vi "Slit.vi"(8 "error in (no error)":errorcluster, 10 "Notifiers":T1, 11 "All Message Queue Cluster":T2) -> (0 "error out":errorcluster)   [LabVIEW 2013]
doc: "Ce VI est la partie visualisation des Fentes. Elle permet l'envoie d'ordre à cette appareil et affiche son état.\n- Connected : indique si l'appareil est connecté.\n- Open : indique l'ouverture de la fente.\n- Status : indique le status actuel de la fente. CAD s'il y a une erreur, ou si elle est en mouvement, etc ..."
uses:
  Lib QMH/AllMessageQueue Cluster.ctl
  Lib QMH/Message Cluster.ctl
  Lib Notifier/Notifier.ctl
  Slit UI data.ctl
  Slit config.ctl
  FGV/Action Slit.ctl
  FGV/FGV Slit Data.ctl
  Lib IHM Control/Front Panel Status.ctl
  support/Status.vi
  Lib QMH/MessageQueues.lvlib
  Lib IHM Control/IHM Control.lvlib
  Lib Notifier/Notifier.lvlib
panel:
  out "Opening":dbl format="%#_3g"
  out "Connected":bool
  out "Status":string
  # "Slit"
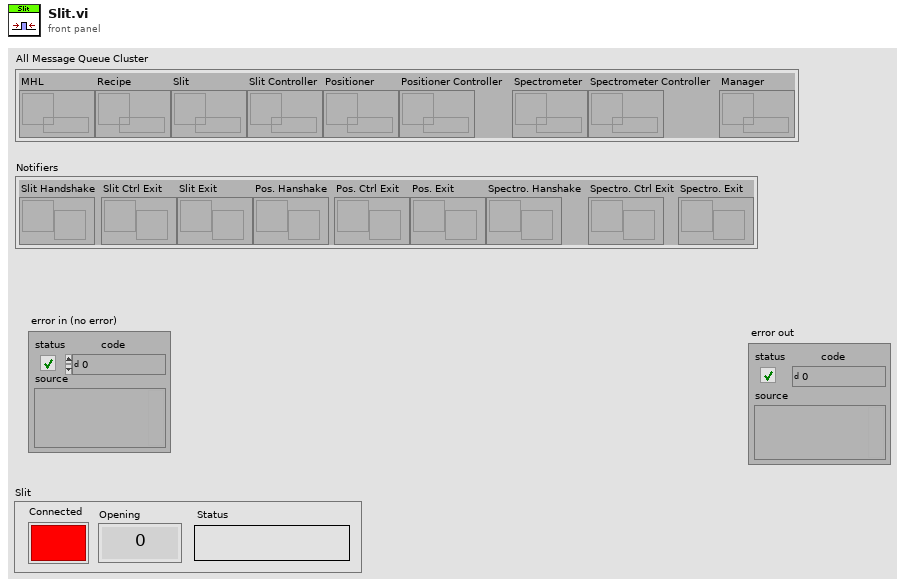
[diagram p1: front panel]
types:
  T1 = typedef "Notifier.lvlib/Notifier.ctl" = cluster{"Slit Handshake":refnum<notifier>, "Slit Ctrl Exit":refnum<notifier>, "Slit Exit":refnum<notifier>, "Pos. Hanshake":refnum<notifier>, "Pos. Ctrl Exit":refnum<notifier>, "Pos. Exit":refnum<notifier>, "Spectro. Hanshake":refnum<notifier>, "Spectro. Ctrl Exit":refnum<notifier>, "Spectro. Exit":refnum<notifier>}
  T2 = typedef "MessageQueues.lvlib/AllMessageQueue Cluster.ctl" = cluster{"MHL":refnum<queue>, "Recipe":refnum<queue>, "Slit":refnum<queue>, "Slit Controller":refnum<queue>, "Positioner":refnum<queue>, "Positioner Controller":refnum<queue>, "Spectrometer":refnum<queue>, "Spectrometer Controller":refnum<queue>, "Manager":refnum<queue>}
  T3 = typedef "Slit config.ctl" = cluster{"VISA resource name":refnum<visa-resource-name>}
  T4 = typedef "Slit UI data.ctl" = cluster{"Connected":bool, "Status":string, "Openning":dbl}
  T5 = typedef "Action Slit.ctl" = enum16{"Connect", "Initialize", "Set Velocity", "Get Velocity", "Move Rel", "Move Abs", "Position", "Status", "Abort", "Disconnect"}
  T6 = typedef "FGV Slit Data.ctl" = cluster{"Portnumber":i32, "Position":dbl, "Status":string, "Système ID":i32, "Connected axes":string[], "Velocity":dbl, "Stage names":string[], "Device ID out":i32}
  T7 = typedef "IHM Control.lvlib/Front Panel Status.ctl" = enum16{"Initialisation", "Enable Slit", "Enable Positionner", "Enable Spectrometer", "Disable Slit", "Disable Positionner", "Disable Spectrometer"}
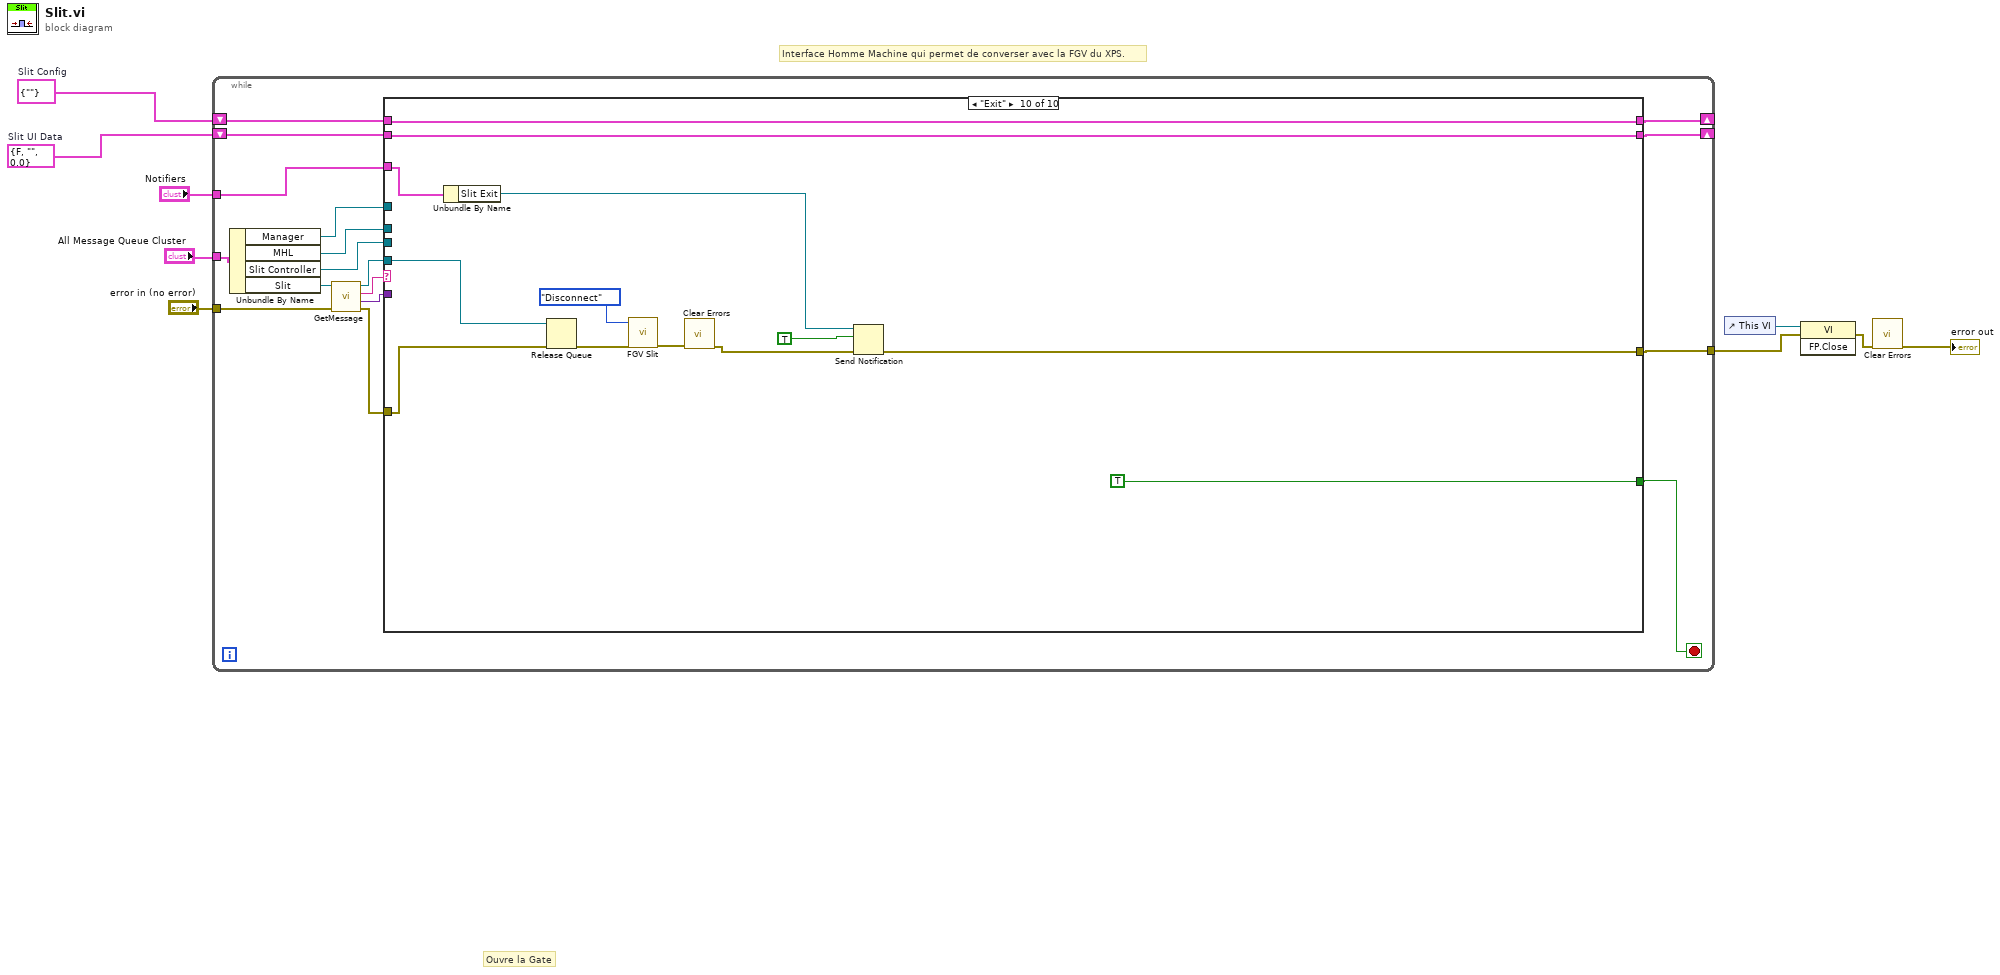
[diagram p0: block diagram]
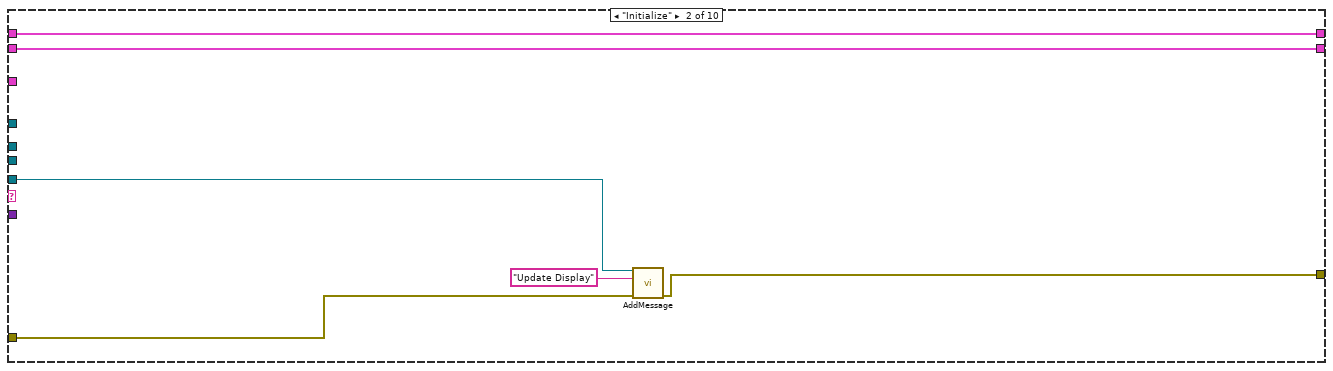
[diagram p3: hidden frame]
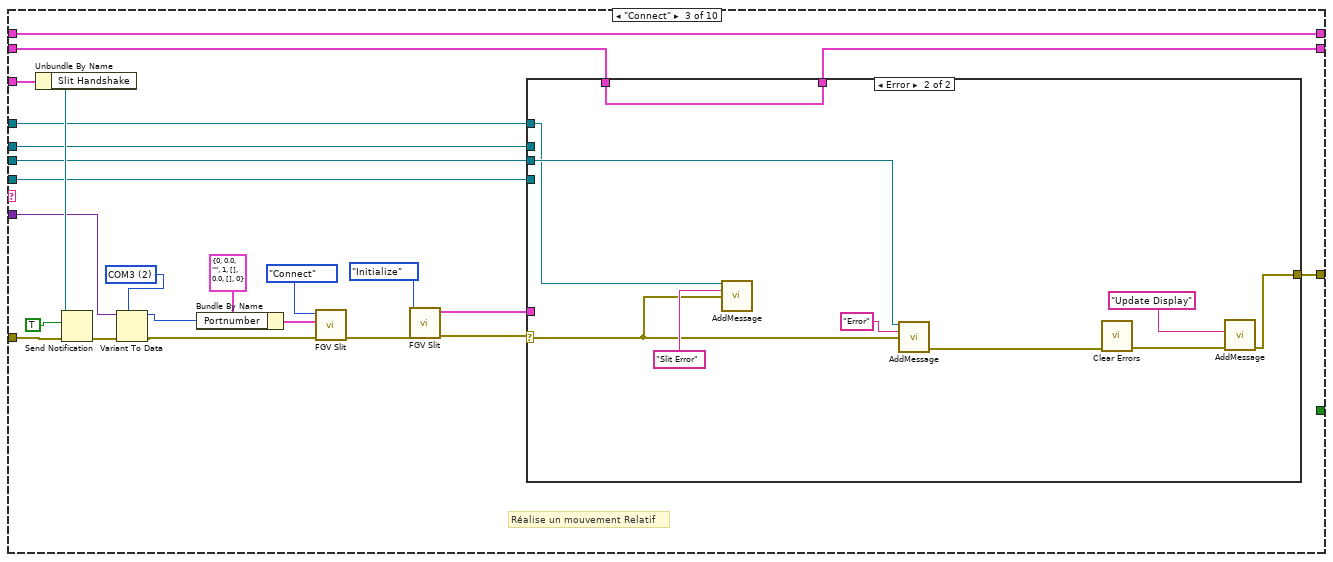
[diagram p4: hidden frame]
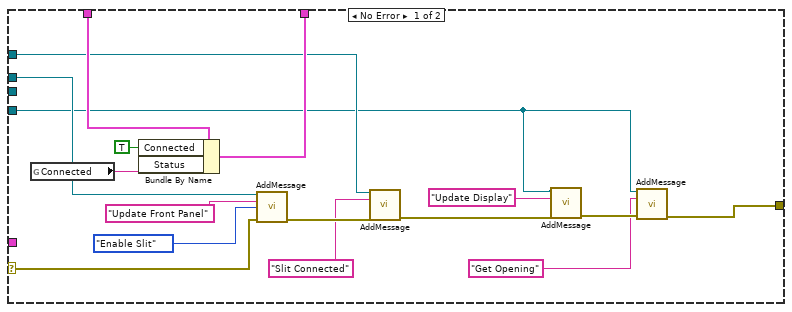
[diagram p5: hidden frame]
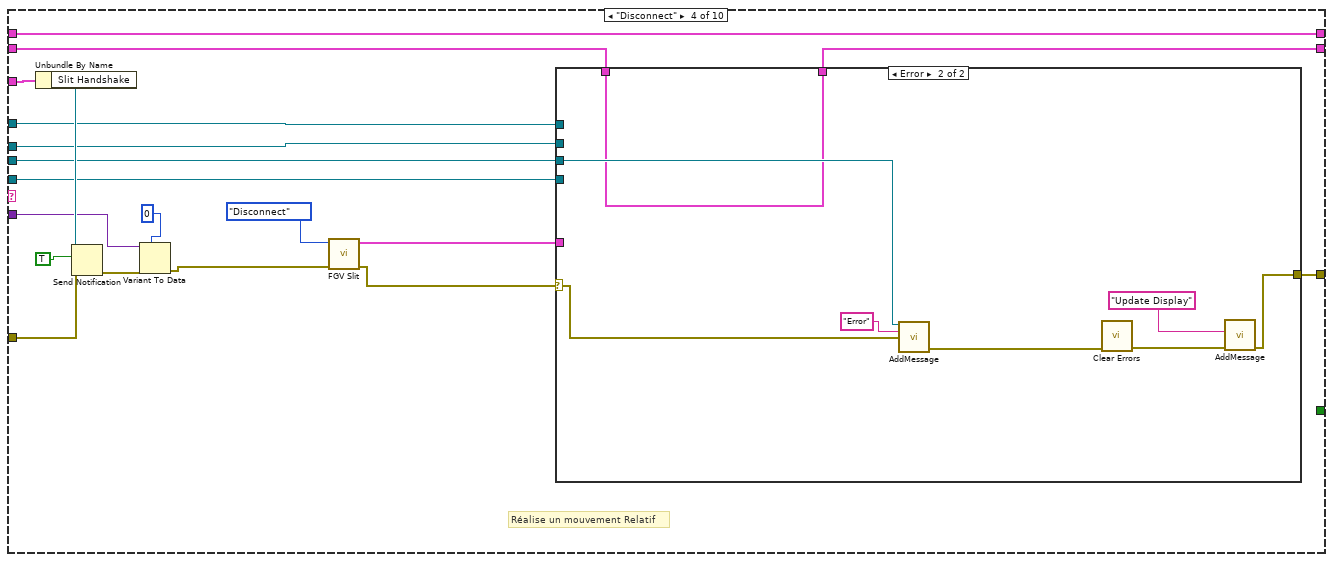
[diagram p6: hidden frame]
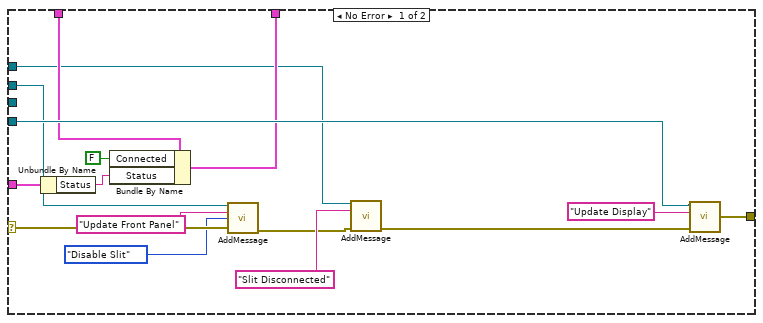
[diagram p7: hidden frame]
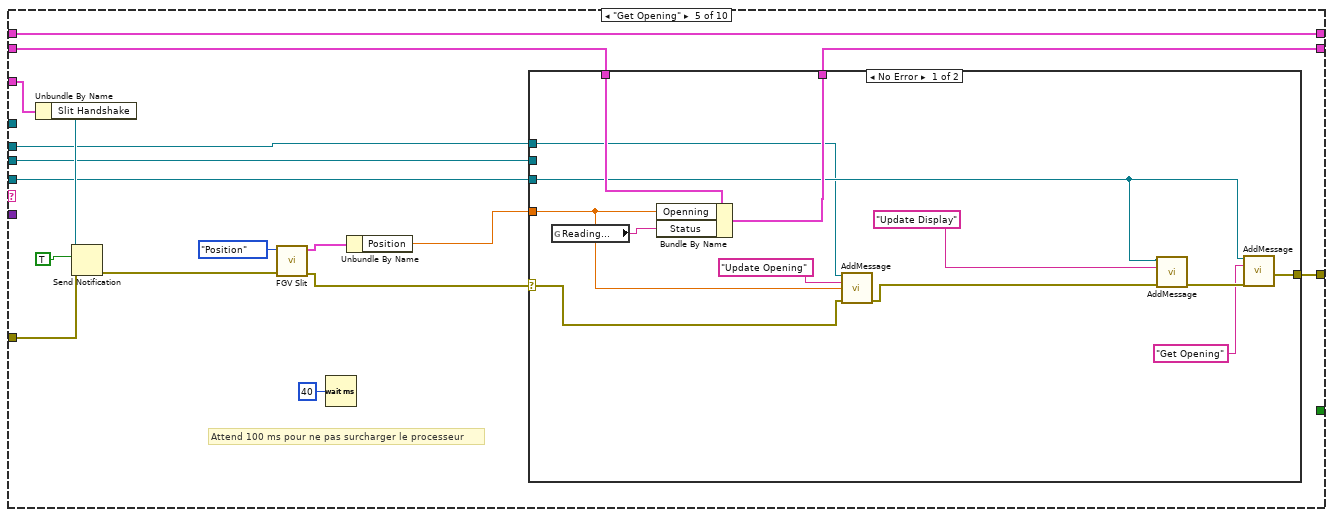
[diagram p8: hidden frame]
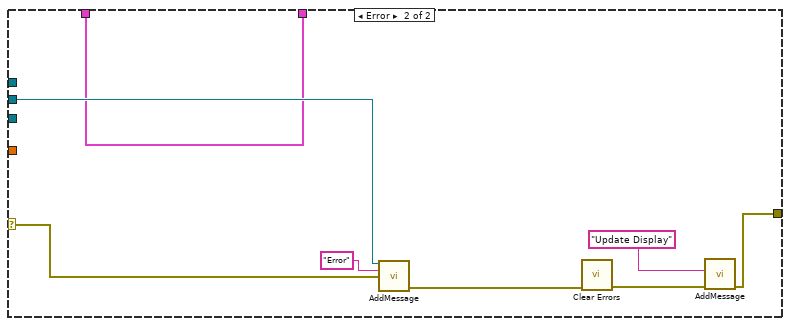
[diagram p9: hidden frame]
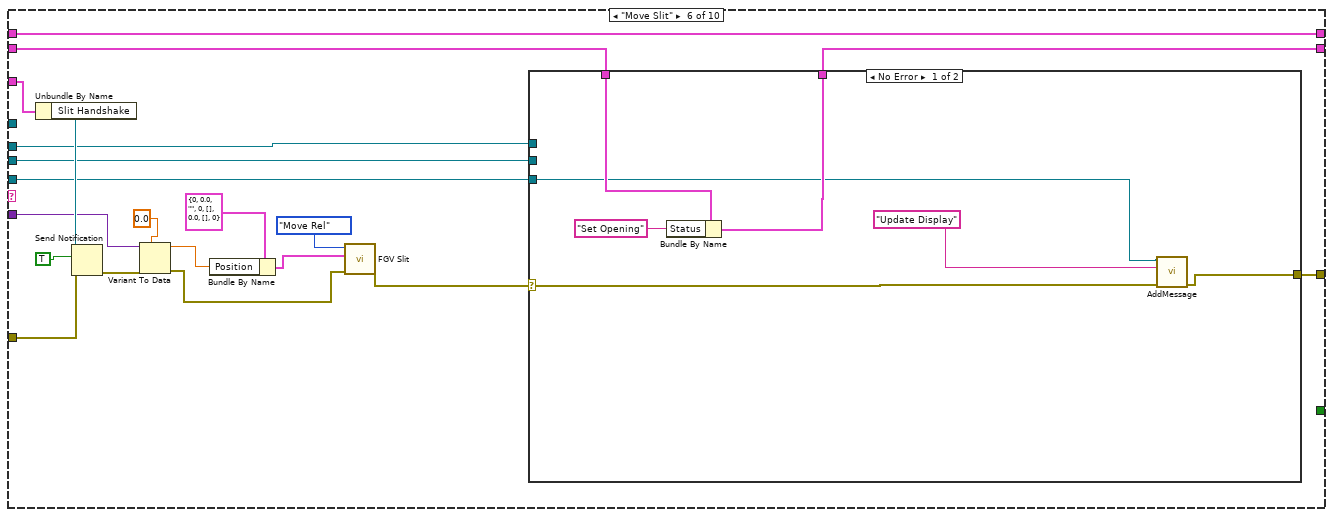
[diagram p10: hidden frame]
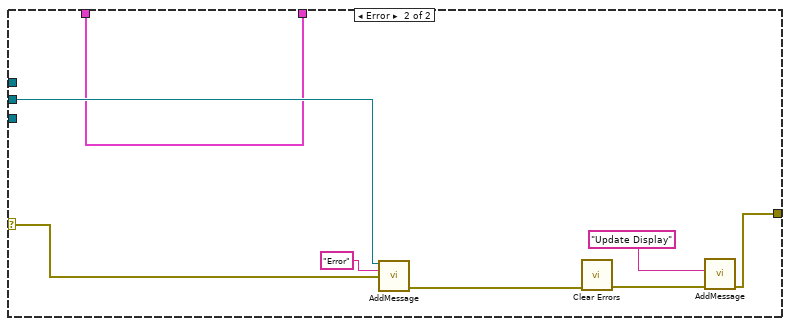
[diagram p11: hidden frame]
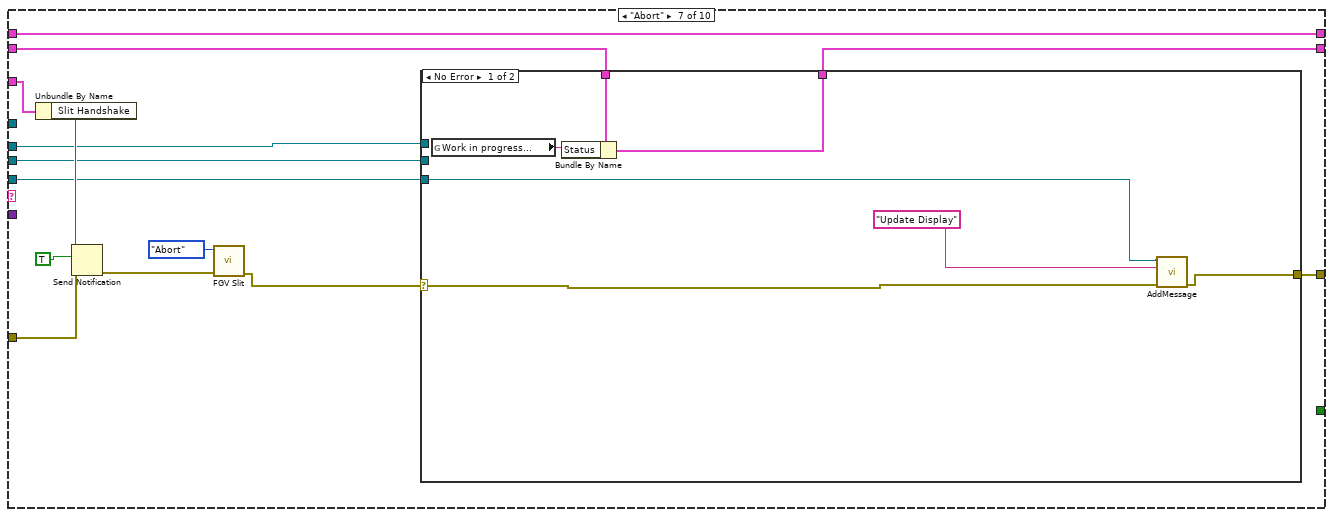
[diagram p12: hidden frame]
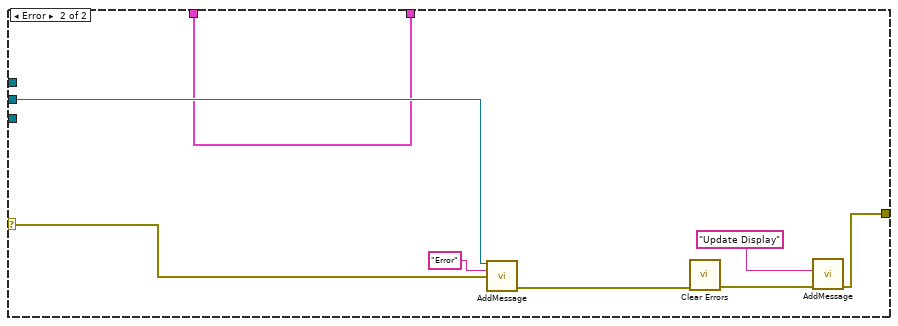
[diagram p13: hidden frame]
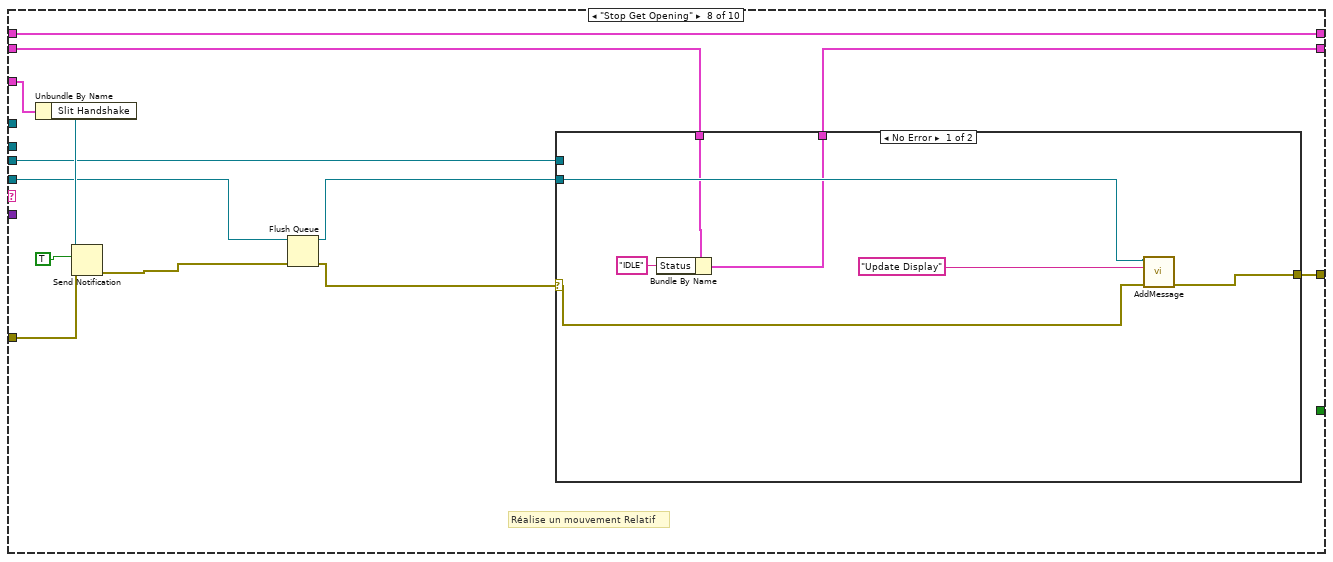
[diagram p14: hidden frame]
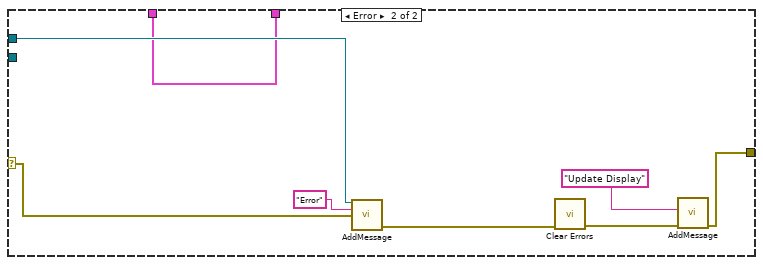
[diagram p15: hidden frame]
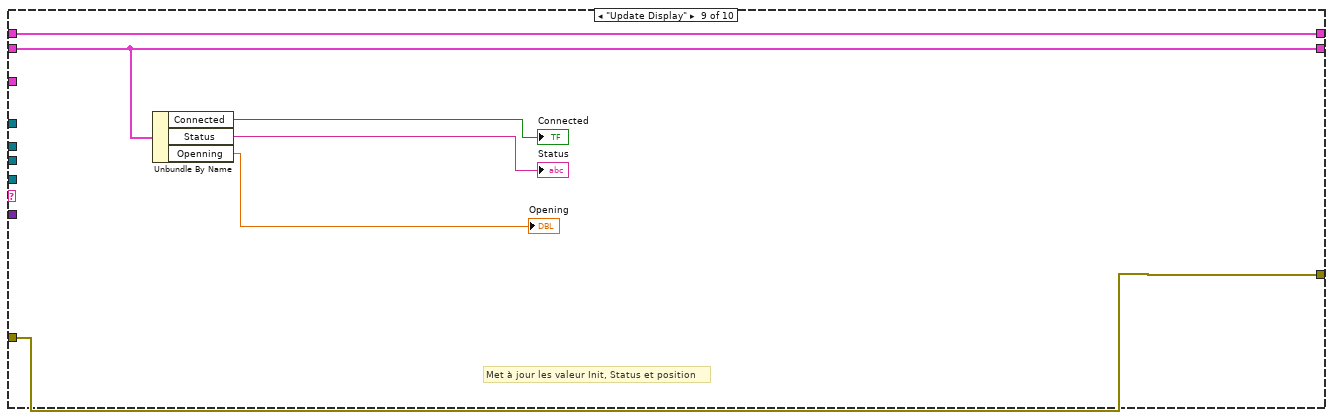
[diagram p16: hidden frame]
diagram:
  w5 = T3 {"VISA resource name"=""}  # Slit Config
  w6 = T4 {"Connected"=FALSE, "Status"="", "Openning"=0.0}  # Slit UI Data
  # "Interface Homme Machine qui permet de converser avec la FGV du XPS."
  # "Ouvre la Gate"
  n1 = while {
    tunnel: "All Message Queue Cluster" -> [w24]
    tunnel: "Notifiers" -> [w17]
    tunnel: "error in (no error)" -> [w25]
    tunnel: [w19] -> w2
    shift-right: [w21] -> _
    shift-left: w5 -> [w23]
    shift-right: [w20] -> _
    shift-left: w6 -> [w22]
    stop <- w18 stop-if-true
    n2 = Unbundle By Name(w24) -> ("Manager"=w16:refnum<queue>, "MHL"=w15:refnum<queue>, "Slit Controller"=w14:refnum<queue>, "Slit"=w26:refnum<queue>)
    n3 = call "GetMessage.vi"("entrée d'erreur"=w25, "Message queue"=w26) -> ("sortie d'erreur"=w12:errorcluster, "Data"=w11:variant, "Message"=w10:string, "Dup Message Queue"=w13:refnum<queue>)  [unwired: 6 in]
    n4 = case shown="\"Exit\"" w10 {
      tunnel: w17 -> [_ _ w57 w103 w144 w185 w214 w242 _ w277]
      tunnel: w13 -> [_ w30 w56 w102 w143 w184 w213 w234 _ w271]
      tunnel: w11 -> [_ _ w43 w94 _ w177 _ _ _ _]
      tunnel: w12 -> [w29 w32 w50 w96 w138 w179 w208 w236 w264 w272]
      tunnel: [w29 w31 w55 w101 w142 w183 w212 w241 w264 w274] -> w19
      tunnel: w14 -> [_ _ w54 w100 w141 w182 w211 w240 _ _]
      tunnel: [_ _ _ _ _ _ _ _ _ TRUE] -> w18
      tunnel: w23 -> [w28 w35 w53 w99 w140 w181 w210 w239 w265 w273]
      tunnel: [w28 w35 w53 w99 w140 w181 w210 w239 w265 w273] -> w21
      tunnel: w22 -> [w27 w34 w52 w98 w135 w174 w206 w238 w263 w270]
      tunnel: [w27 w34 w51 w97 w139 w180 w209 w237 w263 w270] -> w20
      tunnel: w15 -> [_ _ w49 w92 w136 w175 w207 _ _ _]
      tunnel: w16 -> [_ _ w48 w91 _ _ _ _ _ _]
      frame Default {
        # "ne fait rien si le message dépilé n'existe pas"
      }
      frame "Initialize" {
        n5 = call "AddMessage.vi"("Message queue"=w30, "Message"="Update Display", "entrée d'erreur (pas d'erreur)"=w32) -> ("error out"=w31:errorcluster)  [unwired: 11 in, 1 out]
      }
      frame "Connect" {
        w42 = 2 items=["COM1", "COM2", "COM3", "COM4", "COM5", "COM6", "COM7", "COM8", "COM9", "COM10", "COM11", "COM12", "COM13", "COM14", "COM15", "COM16", "COM17", "COM18", "COM19", "COM20", "COM21", "COM22", "COM23", "COM24", "COM25", "COM26", "COM27", "COM28", "COM29", "COM30"] ("Portnumber")
        # "Réalise un mouvement Relatif"
        n6 = Unbundle By Name(w57) -> ("Slit Handshake"=w59:refnum<notifier>)
        n7 = Send Notification(notification=TRUE, notifier=w59, error in (no error)=w50) -> (error out=w44:errorcluster)  [unwired: 1 out]
        n8 = Variant To Data(error in=w44, type=w42, Variant=w43) -> (data=w40:i32, error out=w41:errorcluster)
        n9 = Bundle By Name(cluster=T6 {"Portnumber"=0, "Position"=0.0, "Status"="", "Système ID"=1, "Connected axes"=[], "Velocity"=0.0, "Stage names"=[], "Device ID out"=0} ("FGV Slit Data"), "Portnumber"=w40) -> (w45:T6)
        n10 = call "FGV Slit.vi"("error in (no error)"=w41, "FGV Slit Data In"=w45, "Action"=Action_Slit."Connect") -> ("error out"=w39:errorcluster)  [unwired: 7 in, 1 out]
        n11 = call "FGV Slit.vi"("error in (no error)"=w39, "Action"=Action_Slit."Initialize") -> ("error out"=w38:errorcluster, "FGV Slit Data Out"=w36:T6)  [unwired: 8 in]
        n12 = case shown="Error" w38 {
          selector: w38 -> [w72 w77]
          tunnel: w56 -> [w61 _]
          tunnel: [w62 w82] -> w55
          tunnel: w54 -> [_ w81]
          tunnel: w52 -> [w75 w80]
          tunnel: [w74 w80] -> w51
          tunnel: w49 -> [w71 _]
          tunnel: w48 -> [w66 w78]
          tunnel: w36 -> [_ _]
          frame No Error {
            n13 = global read "Status.vi" "Connected"() -> (w64:string)
            n14 = Bundle By Name(cluster=w75, "Connected"=TRUE, "Status"=w64) -> (w74:T4)
            n15 = call "AddMessage.vi"("Message queue"=w71, "Message"="Update Front Panel", "Data"=Front_Panel_Status."Enable Slit" ("Front Panel status"), "entrée d'erreur (pas d'erreur)"=w72) -> ("error out"=w68:errorcluster)  [unwired: 10 in, 1 out]
            n16 = call "AddMessage.vi"("Message queue"=w66, "Message"="Slit Connected", "entrée d'erreur (pas d'erreur)"=w68) -> ("error out"=w67:errorcluster)  [unwired: 11 in, 1 out]
            n17 = call "AddMessage.vi"("Message queue"=w61, "Message"="Update Display", "entrée d'erreur (pas d'erreur)"=w67) -> ("error out"=w63:errorcluster)  [unwired: 11 in, 1 out]
            n18 = call "AddMessage.vi"("Message queue"=w61, "Message"="Get Opening", "entrée d'erreur (pas d'erreur)"=w63) -> ("error out"=w62:errorcluster)  [unwired: 11 in, 1 out]
          }
          frame Error {
            n19 = call "AddMessage.vi"("Message queue"=w78, "Message"="Slit Error", "Data"=w77) -> ()  [unwired: 11 in, 2 out]
            n20 = call "AddMessage.vi"("Message queue"=w81, "Message"="Error", "Data"=w77) -> ("error out"=w85:errorcluster)  [unwired: 11 in, 1 out]
            n21 = call <vilib>:"Clear Errors.vi"("error in (no error)"=w85) -> ("error out"=w83:errorcluster)  [unwired: 6 in]
            n22 = call "AddMessage.vi"("Message"="Update Display", "entrée d'erreur (pas d'erreur)"=w83) -> ("error out"=w82:errorcluster)  [unwired: 12 in, 1 out]
          }
        }
      }
      frame "Disconnect" {
        # "Réalise un mouvement Relatif"
        n23 = Unbundle By Name(w103) -> ("Slit Handshake"=w105:refnum<notifier>)
        n24 = Send Notification(notification=TRUE, notifier=w105, error in (no error)=w96) -> (error out=w95:errorcluster)  [unwired: 1 out]
        n25 = Variant To Data(error in=w95, type=0, Variant=w94) -> (error out=w90:errorcluster)  [unwired: 1 out]
        n26 = call "FGV Slit.vi"("error in (no error)"=w90, "Action"=Action_Slit."Disconnect") -> ("error out"=w89:errorcluster, "FGV Slit Data Out"=w87:T6)  [unwired: 8 in]
        n27 = case shown="Error" w89 {
          selector: w89 -> [w115 w124]
          tunnel: w102 -> [w121 _]
          tunnel: [w119 w125] -> w101
          tunnel: w100 -> [_ w123]
          tunnel: w98 -> [w118 w122]
          tunnel: [w117 w122] -> w97
          tunnel: w92 -> [w114 _]
          tunnel: w91 -> [w108 _]
          tunnel: w87 -> [w107 _]
          frame No Error {
            n28 = Unbundle By Name(w107) -> ("Status"=w106:string)
            n29 = Bundle By Name(cluster=w118, "Connected"=FALSE, "Status"=w106) -> (w117:T4)
            n30 = call "AddMessage.vi"("Message queue"=w114, "Message"="Update Front Panel", "Data"=Front_Panel_Status."Disable Slit" ("Front Panel status"), "entrée d'erreur (pas d'erreur)"=w115) -> ("error out"=w110:errorcluster)  [unwired: 10 in, 1 out]
            n31 = call "AddMessage.vi"("Message queue"=w108, "Message"="Slit Disconnected", "entrée d'erreur (pas d'erreur)"=w110) -> ("error out"=w109:errorcluster)  [unwired: 11 in, 1 out]
            n32 = call "AddMessage.vi"("Message queue"=w121, "Message"="Update Display", "entrée d'erreur (pas d'erreur)"=w109) -> ("error out"=w119:errorcluster)  [unwired: 11 in, 1 out]
          }
          frame Error {
            n33 = call "AddMessage.vi"("Message queue"=w123, "Message"="Error", "Data"=w124) -> ("error out"=w128:errorcluster)  [unwired: 11 in, 1 out]
            n34 = call <vilib>:"Clear Errors.vi"("error in (no error)"=w128) -> ("error out"=w126:errorcluster)  [unwired: 6 in]
            n35 = call "AddMessage.vi"("Message"="Update Display", "entrée d'erreur (pas d'erreur)"=w126) -> ("error out"=w125:errorcluster)  [unwired: 12 in, 1 out]
          }
        }
      }
      frame "Get Opening" {
        # "Attend 100 ms pour ne pas surcharger le processeur"
        n36 = Unbundle By Name(w144) -> ("Slit Handshake"=w146:refnum<notifier>)
        n37 = Send Notification(notification=TRUE, notifier=w146, error in (no error)=w138) -> (error out=w134:errorcluster)  [unwired: 1 out]
        n38 = call "FGV Slit.vi"("error in (no error)"=w134, "Action"=Action_Slit."Position") -> ("error out"=w133:errorcluster, "FGV Slit Data Out"=w131:T6)  [unwired: 8 in]
        n39 = Wait (ms)(milliseconds to wait=u32 40) -> ()  [unwired: 1 out]
        n40 = Unbundle By Name(w131) -> ("Position"=w130:dbl)
        n41 = case shown="No Error" w133 {
          selector: w133 -> [w152 w162]
          tunnel: w143 -> [w154 _]
          tunnel: [w155 w163] -> w142
          tunnel: w141 -> [_ w161]
          tunnel: w135 -> [w158 w160]
          tunnel: [w157 w160] -> w139
          tunnel: w136 -> [w150 _]
          tunnel: w130 -> [w148 _]
          frame No Error {
            n42 = global read "Status.vi" "Reading..."() -> (w147:string)
            n43 = Bundle By Name(cluster=w158, "Openning"=w148, "Status"=w147) -> (w157:T4)
            n44 = call "AddMessage.vi"("Message queue"=w150, "Message"="Update Opening", "Data"=w148, "entrée d'erreur (pas d'erreur)"=w152) -> ("error out"=w151:errorcluster)  [unwired: 10 in, 1 out]
            n45 = call "AddMessage.vi"("Message queue"=w154, "Message"="Update Display", "entrée d'erreur (pas d'erreur)"=w151) -> ("error out"=w156:errorcluster)  [unwired: 11 in, 1 out]
            n46 = call "AddMessage.vi"("Message queue"=w154, "Message"="Get Opening", "entrée d'erreur (pas d'erreur)"=w156) -> ("error out"=w155:errorcluster)  [unwired: 11 in, 1 out]
          }
          frame Error {
            n47 = call "AddMessage.vi"("Message queue"=w161, "Message"="Error", "Data"=w162) -> ("error out"=w166:errorcluster)  [unwired: 11 in, 1 out]
            n48 = call <vilib>:"Clear Errors.vi"("error in (no error)"=w166) -> ("error out"=w164:errorcluster)  [unwired: 6 in]
            n49 = call "AddMessage.vi"("Message"="Update Display", "entrée d'erreur (pas d'erreur)"=w164) -> ("error out"=w163:errorcluster)  [unwired: 12 in, 1 out]
          }
        }
      }
      frame "Move Slit" {
        n50 = Unbundle By Name(w185) -> ("Slit Handshake"=w187:refnum<notifier>)
        n51 = Send Notification(notification=TRUE, notifier=w187, error in (no error)=w179) -> (error out=w178:errorcluster)  [unwired: 1 out]
        n52 = Variant To Data(error in=w178, type=0.0, Variant=w177) -> (data=w169:dbl, error out=w173:errorcluster)
        n53 = Bundle By Name(cluster=T6 {"Portnumber"=0, "Position"=0.0, "Status"="", "Système ID"=0, "Connected axes"=[], "Velocity"=0.0, "Stage names"=[], "Device ID out"=0} ("FGV Slit Data In"), "Position"=w169) -> (w168:T6)
        n54 = call "FGV Slit.vi"("error in (no error)"=w173, "FGV Slit Data In"=w168, "Action"=Action_Slit."Move Rel") -> ("error out"=w172:errorcluster)  [unwired: 7 in, 1 out]
        n55 = case shown="No Error" w172 {
          selector: w172 -> [w189 w197]
          tunnel: w184 -> [w191 _]
          tunnel: [w188 w198] -> w183
          tunnel: w182 -> [_ w196]
          tunnel: w174 -> [w193 w195]
          tunnel: [w192 w195] -> w180
          tunnel: w175 -> [_ _]
          frame No Error {
            n56 = Bundle By Name(cluster=w193, "Status"="Set Opening") -> (w192:T4)
            n57 = call "AddMessage.vi"("Message queue"=w191, "Message"="Update Display", "entrée d'erreur (pas d'erreur)"=w189) -> ("error out"=w188:errorcluster)  [unwired: 11 in, 1 out]
          }
          frame Error {
            n58 = call "AddMessage.vi"("Message queue"=w196, "Message"="Error", "Data"=w197) -> ("error out"=w201:errorcluster)  [unwired: 11 in, 1 out]
            n59 = call <vilib>:"Clear Errors.vi"("error in (no error)"=w201) -> ("error out"=w199:errorcluster)  [unwired: 6 in]
            n60 = call "AddMessage.vi"("Message"="Update Display", "entrée d'erreur (pas d'erreur)"=w199) -> ("error out"=w198:errorcluster)  [unwired: 12 in, 1 out]
          }
        }
      }
      frame "Abort" {
        n61 = Unbundle By Name(w214) -> ("Slit Handshake"=w216:refnum<notifier>)
        n62 = Send Notification(notification=TRUE, notifier=w216, error in (no error)=w208) -> (error out=w205:errorcluster)  [unwired: 1 out]
        n63 = call "FGV Slit.vi"("error in (no error)"=w205, "Action"=Action_Slit."Abort") -> ("error out"=w204:errorcluster)  [unwired: 8 in, 1 out]
        n64 = case shown="No Error" w204 {
          selector: w204 -> [w221 w226]
          tunnel: w213 -> [w222 _]
          tunnel: [w220 w227] -> w212
          tunnel: w211 -> [_ w225]
          tunnel: w206 -> [w219 w224]
          tunnel: [w218 w224] -> w209
          tunnel: w207 -> [_ _]
          frame No Error {
            n65 = global read "Status.vi" "Work in progress..."() -> (w217:string)
            n66 = Bundle By Name(cluster=w219, "Status"=w217) -> (w218:T4)
            n67 = call "AddMessage.vi"("Message queue"=w222, "Message"="Update Display", "entrée d'erreur (pas d'erreur)"=w221) -> ("error out"=w220:errorcluster)  [unwired: 11 in, 1 out]
          }
          frame Error {
            n68 = call "AddMessage.vi"("Message queue"=w225, "Message"="Error", "Data"=w226) -> ("error out"=w230:errorcluster)  [unwired: 11 in, 1 out]
            n69 = call <vilib>:"Clear Errors.vi"("error in (no error)"=w230) -> ("error out"=w228:errorcluster)  [unwired: 6 in]
            n70 = call "AddMessage.vi"("Message"="Update Display", "entrée d'erreur (pas d'erreur)"=w228) -> ("error out"=w227:errorcluster)  [unwired: 12 in, 1 out]
          }
        }
      }
      frame "Stop Get Opening" {
        # "Réalise un mouvement Relatif"
        n71 = Unbundle By Name(w242) -> ("Slit Handshake"=w244:refnum<notifier>)
        n72 = Send Notification(notification=TRUE, notifier=w244, error in (no error)=w236) -> (error out=w232:errorcluster)  [unwired: 1 out]
        n73 = Flush Queue(queue=w234, error in (no error)=w232) -> (queue out=w233:refnum<queue>, error out=w235:errorcluster)  [unwired: 1 out]
        n74 = case shown="No Error" w235 {
          selector: w235 -> [w248 w254]
          tunnel: w233 -> [w251 _]
          tunnel: [w249 w255] -> w241
          tunnel: w240 -> [_ w253]
          tunnel: w238 -> [w247 w252]
          tunnel: [w245 w252] -> w237
          frame No Error {
            n75 = Bundle By Name(cluster=w247, "Status"="IDLE") -> (w245:T4)
            n76 = call "AddMessage.vi"("Message queue"=w251, "Message"="Update Display", "entrée d'erreur (pas d'erreur)"=w248) -> ("error out"=w249:errorcluster)  [unwired: 11 in, 1 out]
          }
          frame Error {
            n77 = call "AddMessage.vi"("Message queue"=w253, "Message"="Error", "Data"=w254) -> ("error out"=w258:errorcluster)  [unwired: 11 in, 1 out]
            n78 = call <vilib>:"Clear Errors.vi"("error in (no error)"=w258) -> ("error out"=w256:errorcluster)  [unwired: 6 in]
            n79 = call "AddMessage.vi"("Message"="Update Display", "entrée d'erreur (pas d'erreur)"=w256) -> ("error out"=w255:errorcluster)  [unwired: 12 in, 1 out]
          }
        }
      }
      frame "Update Display" {
        # "Met à jour les valeur Init, Status et position"
        n80 = Unbundle By Name(w263) -> ("Connected"=→"Connected":bool, "Status"=→"Status":string, "Openning"=→"Opening":dbl)
      }
      frame "Exit" {
        n81 = Unbundle By Name(w277) -> ("Slit Exit"=w276:refnum<notifier>)
        n82 = Release Queue(queue=w271, error in (no error)=w272) -> (error out=w268:errorcluster)  [unwired: 1 in, 2 out]
        n83 = call "FGV Slit.vi"("error in (no error)"=w268, "Action"=Action_Slit."Disconnect") -> ("error out"=w267:errorcluster)  [unwired: 8 in, 1 out]
        n84 = call <vilib>:"Clear Errors.vi"("error in (no error)"=w267) -> ("error out"=w266:errorcluster)  [unwired: 6 in]
        n85 = Send Notification(notification=TRUE, notifier=w276, error in (no error)=w266) -> (error out=w274:errorcluster)  [unwired: 1 out]
      }
    }
  }
  n86 = control-ref of="This VI"() -> (w4:refnum<vi>)
  n87 = invoke class="VI" method="FP.Close"(reference=w4, error in=w2) -> (error out=w3:errorcluster)  [unwired: 1 in, 2 out]
  n88 = call <vilib>:"Clear Errors.vi"("error in (no error)"=w3) -> ("error out"=→"error out":errorcluster)  [unwired: 6 in]
